vi "Init.vi"(8 "error in (no error)":errorcluster, 11 "Carya Config (By Reference)":refnum<class "Carya Config (By Reference).lvclass">) -> (0 "error out":errorcluster, 3 "Carya Config (Buffer) out":refnum<class "CConfig Nonpersistant Buffer.lvclass">)   [LabVIEW 2013, in "CConfig Nonpersistant Buffer.lvclass"]
doc: "Copyright 2018, Carya Automatisering, Wiebe Walstra."
uses:
  CConfig Nonpersistant Buffer.lvclass
  Carya Config (By Reference).lvclass
  Carya Config.lvclass
  CConfig Nonpersistant Buffer.lvclass/CConfig Nonpersistant Buffer.ctl
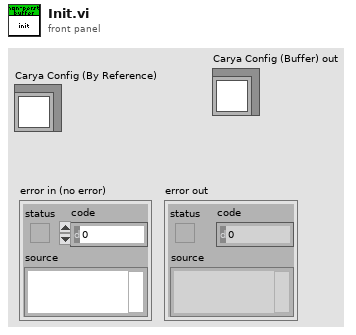
[diagram p1: front panel]
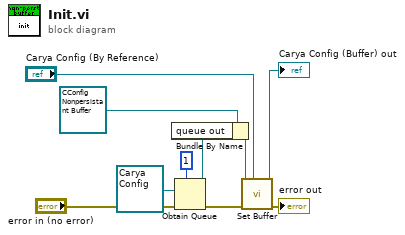
[diagram p0: block diagram]
diagram:
  n1 = Obtain Queue(max queue size (-1, unlimited)=1, element data type=refnum<class "Carya Config.lvclass"> refnum ("Carya Config.lvclass"), error in (no error)="error in (no error)") -> (queue out=w8:refnum<queue>, error out=w7:errorcluster)  [unwired: 2 in, 1 out]
  n2 = Bundle By Name(cluster=refnum<class "CConfig Nonpersistant Buffer.lvclass"> refnum ("Carya Config (Buffer) in"), "queue out"=w8) -> (w4:refnum<class "CConfig Nonpersistant Buffer.lvclass">)
  n3 = call-dynamic "Set Buffer.vi"("Config in"="Carya Config (By Reference)", "error in (no error)"=w7, "Carya Config (Buffer) in"=w4) -> ("error out"=→"error out":errorcluster, "Carya Config (Buffer) out"=→"Carya Config (Buffer) out":refnum<class "CConfig Nonpersistant Buffer.lvclass">)  [unwired: 6 in, 1 out]
